vi "HRM-GUI-main-test.vi"(8 "error in (no error)":errorcluster, 11 "init cluster":T1) -> (0 "error out":errorcluster)   [LabVIEW 2020]
uses:
  init/HRM-init-cluster.ctl
  init/HRM-init-user_events.ctl
  process/HRM-process-Pulse settings.ctl
  init/HRM-init-Intial State.ctl
  init/HRM-init-hardware_selector.ctl
panel:
  in  "Manual?":bool
  in  "bottom":dbl
  in  "Top":dbl
  in  "Tab Control":enum32{"Raw collected data", "Filtered data"}(tab)
  out "Raw collected data":waveform(dbl)(graph)
  out "Filtered data":waveform(dbl)(graph)
  in  "Clear stored waveform":bool
  in  "Pause AQN":bool
  out "Status Feedback":string
  in  "Additional Signal to remove [s]":i32
  in  "samples [s]":i32=10
  in  "stop":bool
  out "Heart Rate":dbl format="%.2p"
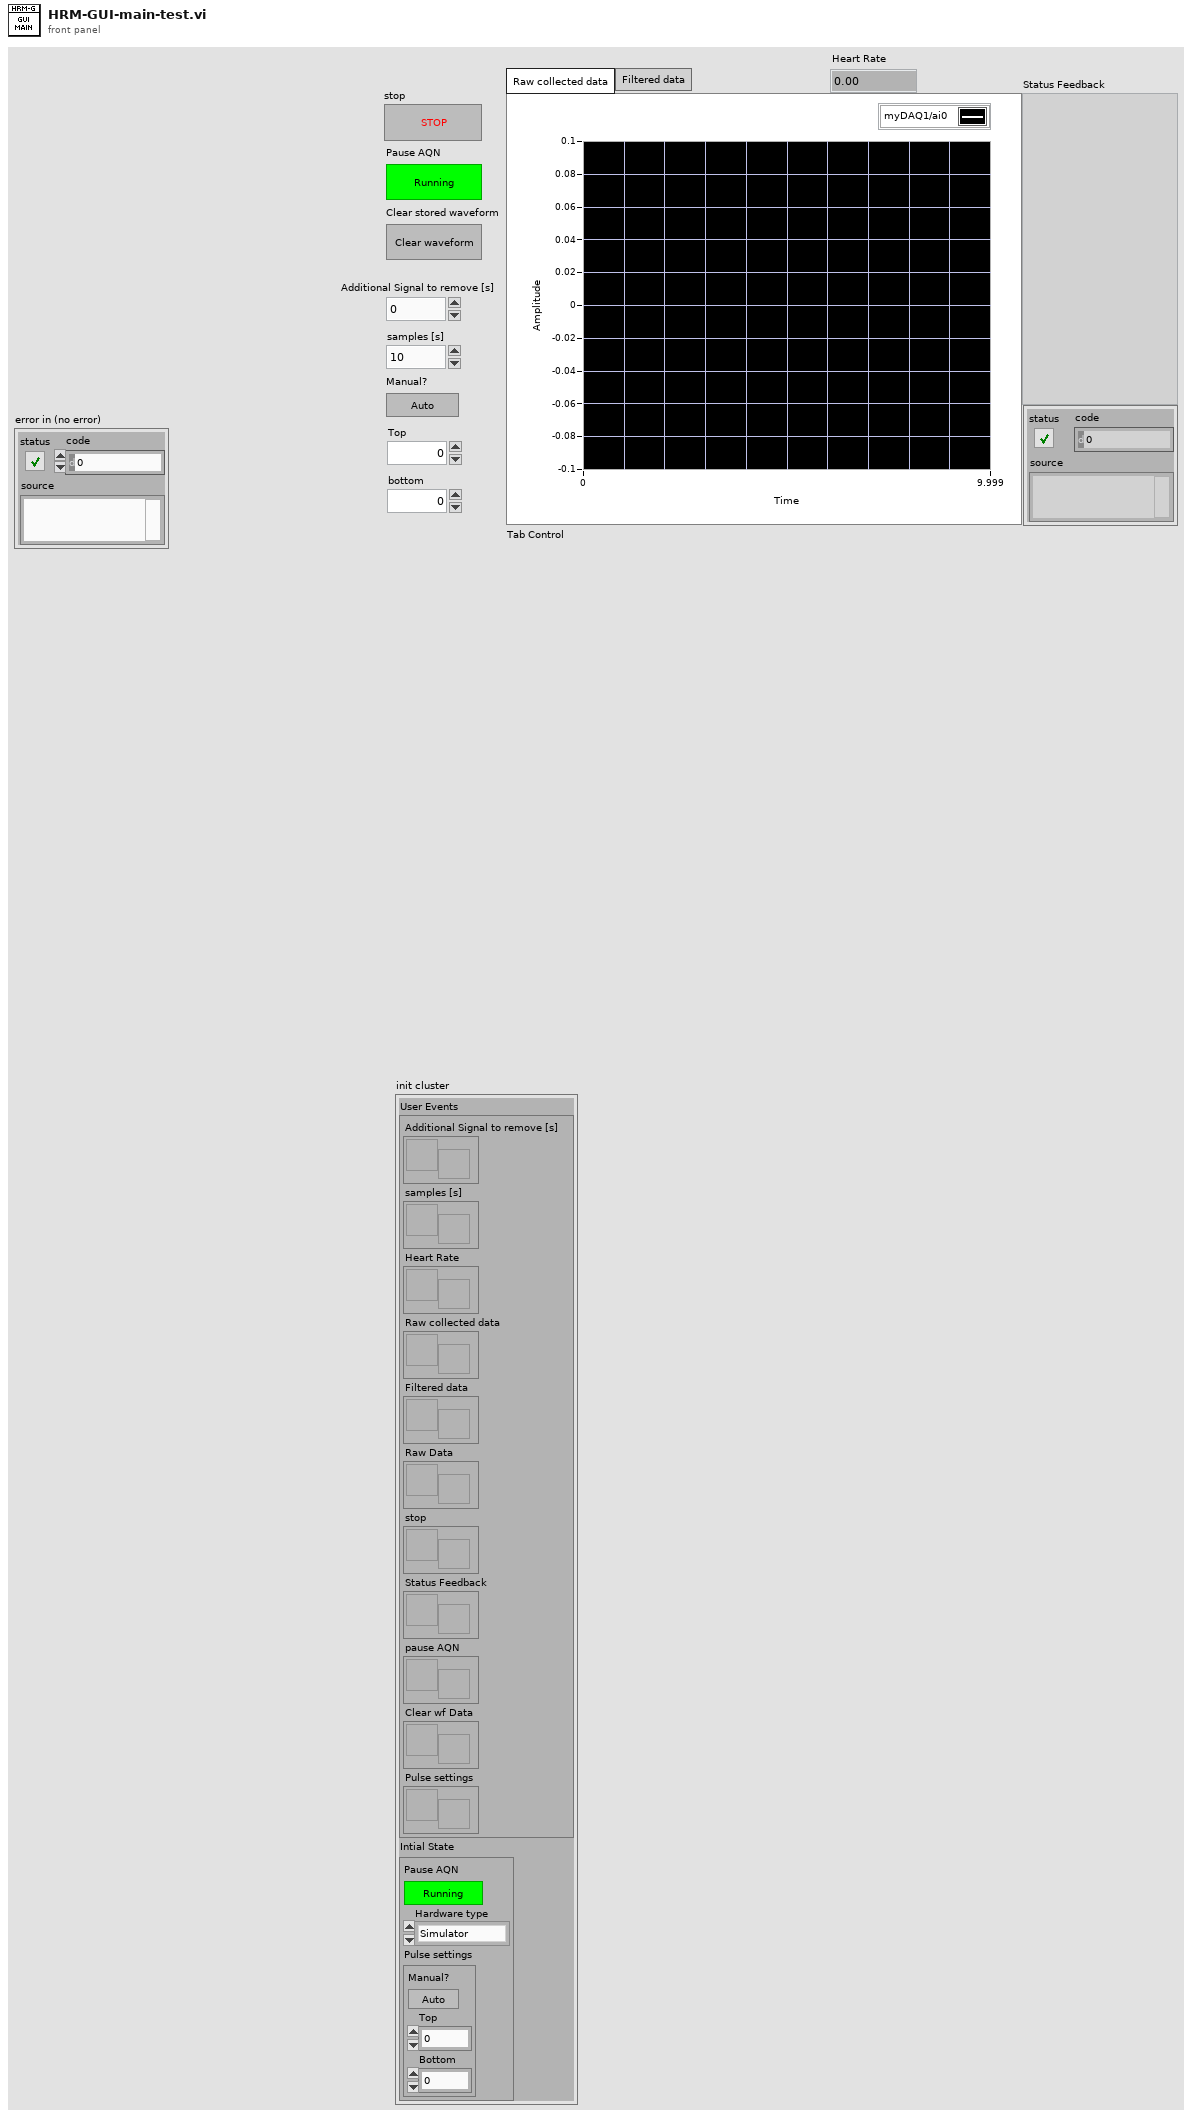
[diagram p1: front panel]
types:
  T1 = typedef "HRM-init-cluster.ctl" = cluster{"User Events":T2, "Intial State":T3}
  T2 = typedef "HRM-init-user_events.ctl" = cluster{"Additional Signal to remove [s]":refnum<user-event>, "samples [s]":refnum<user-event>, "Heart Rate":refnum<user-event>, "Raw collected data":refnum<user-event>, "Filtered data":refnum<user-event>, "Raw Data":refnum<user-event>, "stop":refnum<user-event>, "Status Feedback":refnum<user-event>, "pause AQN":refnum<user-event>, "Clear wf Data":refnum<user-event>, "Pulse settings":refnum<user-event>}
  T3 = typedef "HRM-init-Intial State.ctl" = cluster{"Pause AQN":bool, "Hardware type":T4, "Pulse settings":T5}
  T4 = typedef "HRM-init-hardware_selector.ctl" = enum16{"Simulator", "myDAQ", "Arduino", "Analog Discovery"}
  T5 = typedef "HRM-process-Pulse settings.ctl" = cluster{"Manual?":bool, "Top":dbl, "Bottom":dbl}
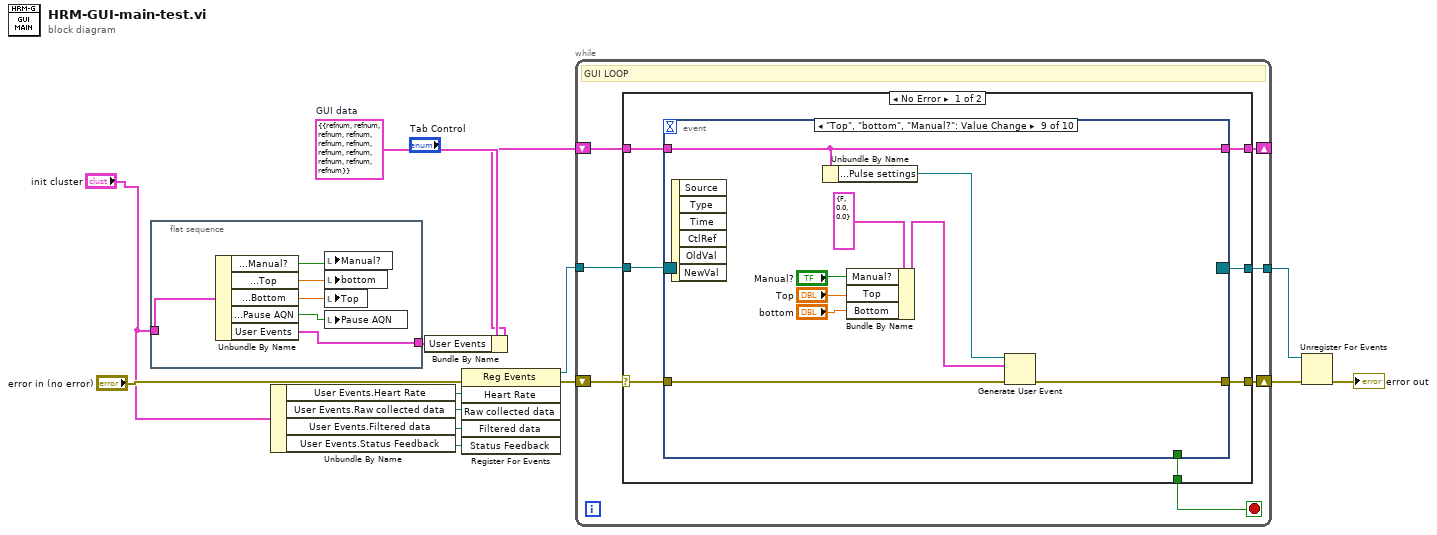
[diagram p0: block diagram]
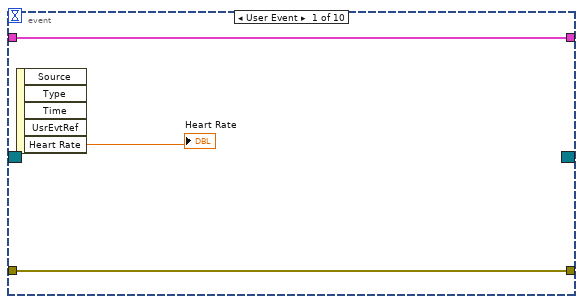
[diagram p2: hidden frame]
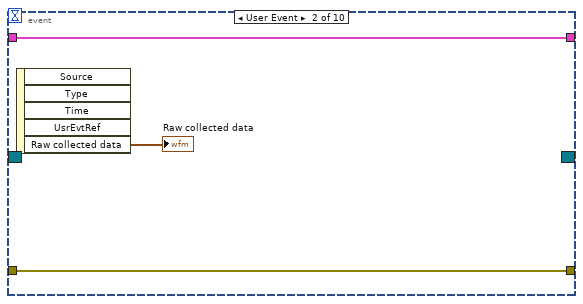
[diagram p3: hidden frame]
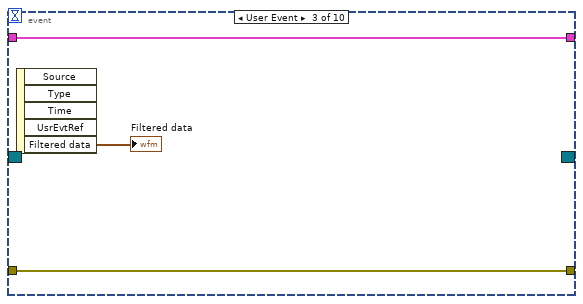
[diagram p4: hidden frame]
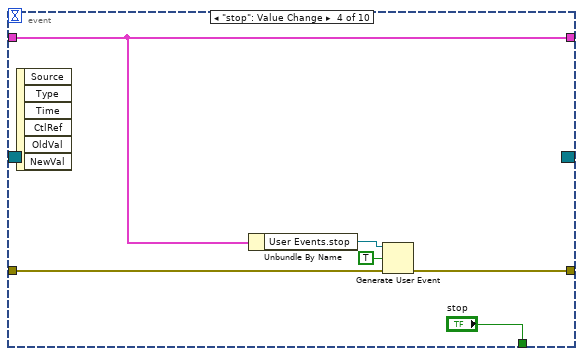
[diagram p5: hidden frame]
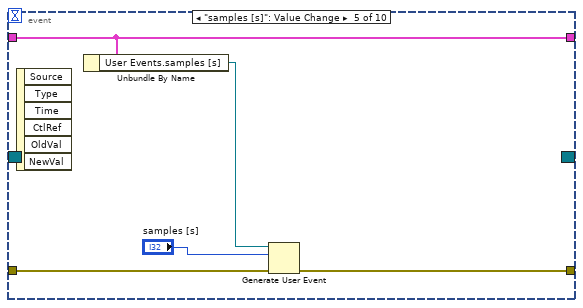
[diagram p6: hidden frame]
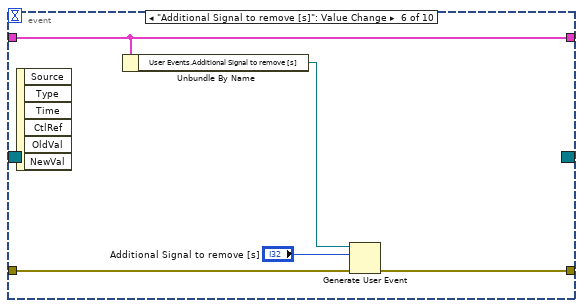
[diagram p7: hidden frame]
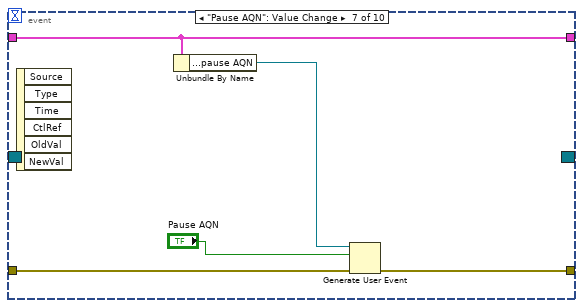
[diagram p8: hidden frame]
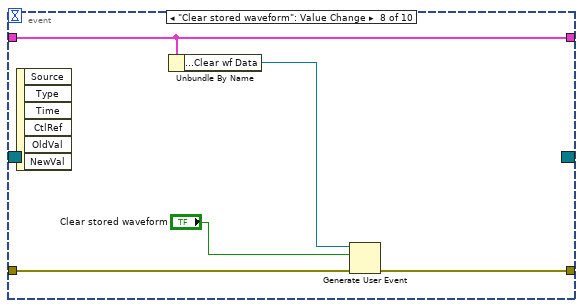
[diagram p9: hidden frame]
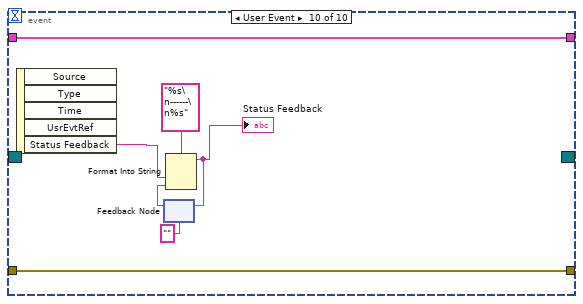
[diagram p10: hidden frame]
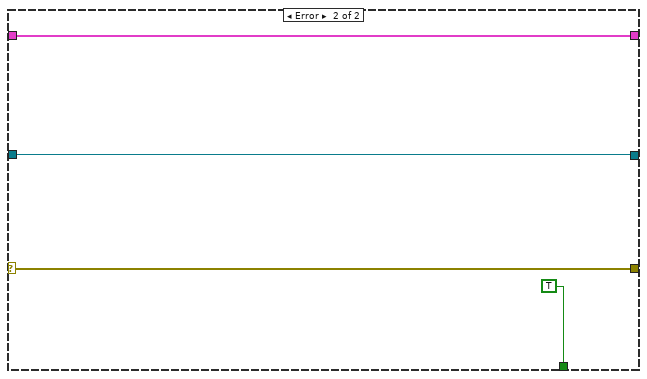
[diagram p11: hidden frame]
diagram:
  w9 = cluster{"User Events":T2} {"User Events"={"Additional Signal to remove [s]"=refnum, "samples [s]"=refnum, "Heart Rate"=refnum, "Raw collected data"=refnum, "Filtered data"=refnum, "Raw Data"=refnum, "stop"=refnum, "Status Feedback"=refnum, "pause AQN"=refnum, "Clear wf Data"=refnum, "Pulse settings"=refnum}}  # GUI data
  n1 = flat-sequence {
    tunnel: [w20] -> w7
    tunnel: "init cluster" -> [w19]
    frame #0 {
      n2 = Unbundle By Name(w19) -> ("Intial State.Pulse settings.Manual?"=w17:bool, "Intial State.Pulse settings.Top"=w16:dbl, "Intial State.Pulse settings.Bottom"=w15:dbl, "Intial State.Pause AQN"=w18:bool, "User Events"=w20:T2)
      n3 = local write "Manual?"(w17) -> ()
      n4 = local write "bottom"(w16) -> ()
      n5 = local write "Top"(w15) -> ()
      n6 = local write "Pause AQN"(w18) -> ()
    }
  }
  n7 = Unbundle By Name("init cluster") -> ("User Events.Heart Rate"=w14:refnum<user-event>, "User Events.Raw collected data"=w6:refnum<user-event>, "User Events.Filtered data"=w5:refnum<user-event>, "User Events.Status Feedback"=w1:refnum<user-event>)
  n8 = Bundle By Name(cluster=w9, "User Events"=w7) -> (w8:cluster{"User Events":T2})
  n9 = register-events(error in="error in (no error)", w14, w6, w5, w1) -> (reference out=w10:refnum<event-registration>, error out=w11:errorcluster)  [unwired: 1 in]
  n10 = while {
    shift-right: [w26] -> w13
    shift-left: w11 -> [w27]
    tunnel: w10 -> [w24]
    tunnel: [w23] -> w12
    shift-right: [w22] -> _
    shift-left: w8 -> [w21]
    stop <- w25 stop-if-true
    # "GUI LOOP"
    n11 = case shown="No Error" w27 {
      selector: w27 -> [w34 w89]
      tunnel: [w29 w89] -> w26
      tunnel: [w28 TRUE] -> w25
      tunnel: w24 -> [w33 w87]
      tunnel: [w32 w87] -> w23
      tunnel: [w31 w86] -> w22
      tunnel: w21 -> [w30 w86]
      frame No Error {
        n12 = event shown="[8] \"Top\", \"bottom\", \"Manual?\": Value Change" {
          selector: w33 -> [_ _ _ _ _ _ _ _ _ _]
          dyn-events: [_ _ _ _ _ _ _ _ _ _] -> w32
          timeout: _ -> [_ _ _ _ _ _ _ _ _ _]
          tunnel: w34 -> [w36 w40 w42 w48 w52 w57 w62 w67 w76 w84]
          tunnel: [w35 w38 w41 w46 w54 w59 w64 w69 w78 w85] -> w31
          tunnel: w30 -> [w35 w38 w41 w46 w54 w59 w64 w69 w78 w85]
          tunnel: [w36 w40 w42 w47 w51 w56 w61 w66 w75 w84] -> w29
          tunnel: [_ _ _ "stop" _ _ _ _ _ _] -> w28
          event User Event {
            n13 = event-data() -> ("Heart Rate"=→"Heart Rate":dbl)  [unwired: 1 in, 4 out]
          }
          event User Event {
            n14 = event-data() -> ("Raw collected data"=→"Raw collected data":waveform(dbl))  [unwired: 1 in, 4 out]
          }
          event User Event {
            n15 = event-data() -> ("Filtered data"=→"Filtered data":waveform(dbl))  [unwired: 1 in, 4 out]
          }
          event "stop": Value Change {
            n16 = event-data() -> ()  [unwired: 1 in, 6 out]
            n17 = Unbundle By Name(w46) -> ("User Events.stop"=w45:refnum<user-event>)
            n18 = Generate User Event(user event=w45, event data cluster=TRUE ("event data"), error in=w48) -> (error out=w47:errorcluster)  [unwired: 1 in, 1 out]
          }
          event "samples [s]": Value Change {
            n19 = event-data() -> ()  [unwired: 1 in, 6 out]
            n20 = Unbundle By Name(w54) -> ("User Events.samples [s]"=w53:refnum<user-event>)
            n21 = Generate User Event(user event=w53, event data cluster="samples [s]", error in=w52) -> (error out=w51:errorcluster)  [unwired: 1 in, 1 out]
          }
          event "Additional Signal to remove [s]": Value Change {
            n22 = event-data() -> ()  [unwired: 1 in, 6 out]
            n23 = Unbundle By Name(w59) -> ("User Events.Additional Signal to remove [s]"=w58:refnum<user-event>)
            n24 = Generate User Event(user event=w58, event data cluster="Additional Signal to remove [s]", error in=w57) -> (error out=w56:errorcluster)  [unwired: 1 in, 1 out]
          }
          event "Pause AQN": Value Change {
            n25 = event-data() -> ()  [unwired: 1 in, 6 out]
            n26 = Unbundle By Name(w64) -> ("User Events.pause AQN"=w63:refnum<user-event>)
            n27 = Generate User Event(user event=w63, event data cluster="Pause AQN", error in=w62) -> (error out=w61:errorcluster)  [unwired: 1 in, 1 out]
          }
          event "Clear stored waveform": Value Change {
            n28 = event-data() -> ()  [unwired: 1 in, 6 out]
            n29 = Unbundle By Name(w69) -> ("User Events.Clear wf Data"=w68:refnum<user-event>)
            n30 = Generate User Event(user event=w68, event data cluster="Clear stored waveform", error in=w67) -> (error out=w66:errorcluster)  [unwired: 1 in, 1 out]
          }
          event "Top", "bottom", "Manual?": Value Change {
            n31 = event-data() -> ()  [unwired: 1 in, 6 out]
            n32 = Unbundle By Name(w78) -> ("User Events.Pulse settings"=w77:refnum<user-event>)
            n33 = Bundle By Name(cluster=T5 {"Manual?"=FALSE, "Top"=0.0, "Bottom"=0.0} ("Pulse settings"), "Manual?"="Manual?", "Top"="Top", "Bottom"="bottom") -> (w73:T5)
            n34 = Generate User Event(user event=w77, event data cluster=w73, error in=w76) -> (error out=w75:errorcluster)  [unwired: 1 in, 1 out]
          }
          event User Event {
            n35 = event-data() -> ("Status Feedback"=w81:string)  [unwired: 1 in, 4 out]
            n36 = feedback #1("") -> (w82:string)
            n37 = Format Into String(format string="%s\n------\n%s", w81, w82) -> (resulting string=w79:string)  [unwired: 2 in, 1 out]
            "Status Feedback" <- w79
            n38 = feedback-in #1(w79) -> ()
          }
        }
      }
      frame Error {
      }
    }
  }
  n39 = Unregister For Events(event registration refnum=w12, error in=w13) -> (error out=→"error out":errorcluster)
